vi "Write Core UI References.vi"(8 "error in (no error)":errorcluster, 10 "UI References":T1, 11 "CIF_UI in":refnum<class "CIF_UI.lvclass">) -> (0 "error out":errorcluster, 3 "CIF_UI out":refnum<class "CIF_UI.lvclass">)   [LabVIEW 2021, in "CIF_UI.lvclass"]
uses:
  CIF_UI.lvclass
  Typedef/Core UI References.ctl
  Typedef/Channel Connection.ctl
  Typedef/New Plugin.ctl
  Typedef/Run Listen Button.ctl
  Typedef/CIF_Manager_UI_Tab.ctl
  CIF_UI.lvclass/CIF_UI.ctl
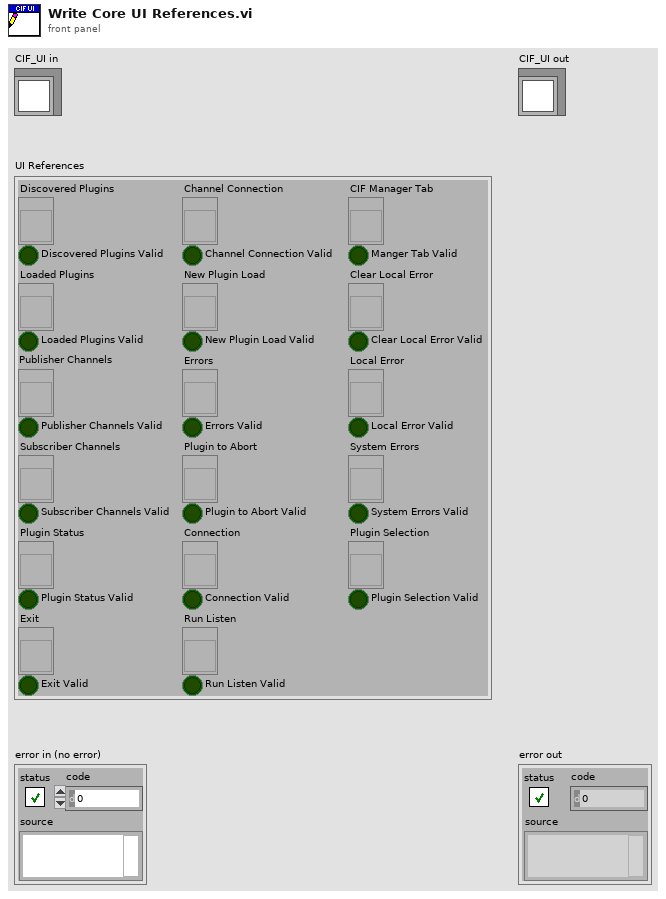
[diagram p1: front panel]
types:
  T1 = typedef "CIF_UI.lvclass/Core UI References.ctl" = cluster{"Discovered Plugins":refnum<vi>, "Discovered Plugins Valid":bool, "Loaded Plugins":refnum<vi>, "Loaded Plugins Valid":bool, "Publisher Channels":refnum<vi>, "Publisher Channels Valid":bool, "Subscriber Channels":refnum<vi>, "Subscriber Channels Valid":bool, "Plugin Status":refnum<vi>, "Plugin Status Valid":bool, "Channel Connection":refnum<vi>, "Channel Connection Valid":bool, "New Plugin Load":refnum<vi>, "New Plugin Load Valid":bool, "Errors":refnum<vi>, "Errors Valid":bool, "Plugin to Abort":refnum<vi>, "Plugin to Abort Valid":bool, "Connection":refnum<vi>, "Connection Valid":bool, "Exit":refnum<vi>, "Exit Valid":bool, "Run Listen":refnum<vi>, "Run Listen Valid":bool, "CIF Manager Tab":refnum<vi>, "Manger Tab Valid":bool, "Clear Local Error":refnum<vi>, "Clear Local Error Valid":bool, "Local Error":refnum<vi>, "Local Error Valid":bool, "System Errors":refnum<vi>, "System Errors Valid":bool, "Plugin Selection":refnum<vi>, "Plugin Selection Valid":bool}
  T2 = typedef "CIF_UI.lvclass/Channel Connection.ctl" = cluster{"Subscriber Name":string, "Publisher Name":string, "Custom Data":string, "FIFO Overrides":cluster{"Backpressure":bool, "Bytes/Message":u32, "Messages/FIFO":u32}}
  T3 = typedef "CIF_UI.lvclass/New Plugin.ctl" = cluster{"Unique Name":string, "Type":string, "Version (Optional)":string}
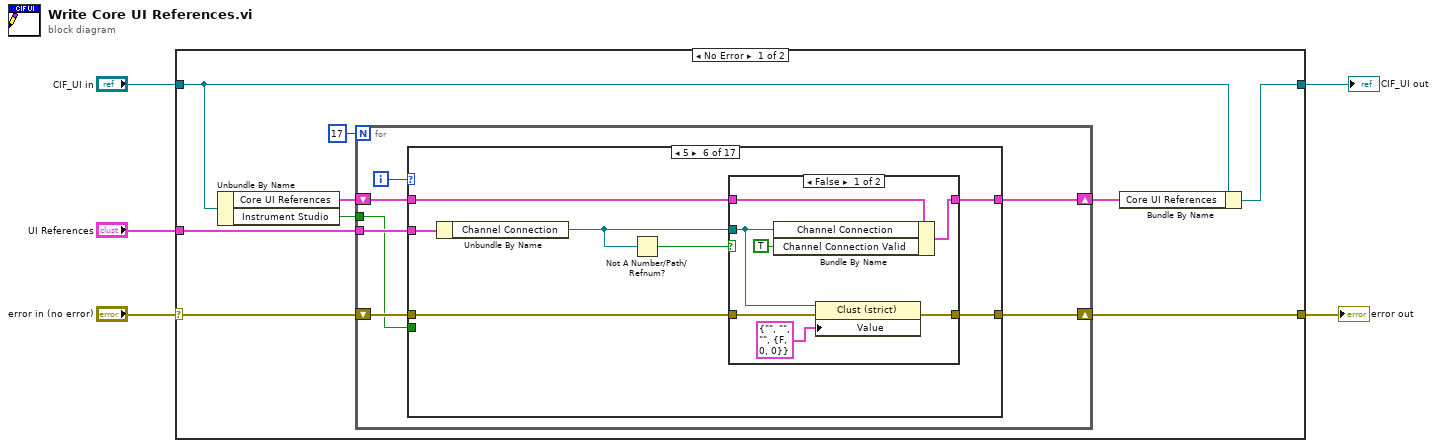
[diagram p0: block diagram]
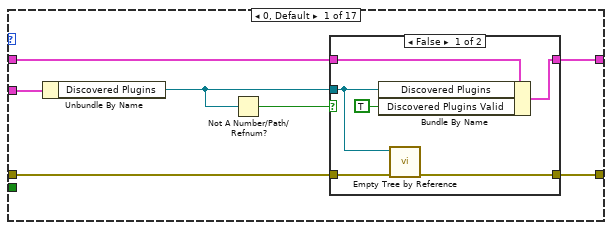
[diagram p2: hidden frame]
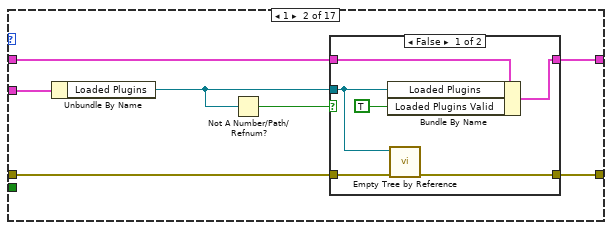
[diagram p4: hidden frame]
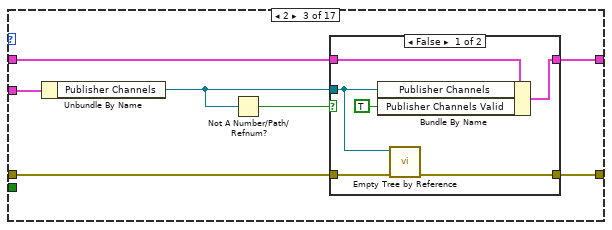
[diagram p6: hidden frame]
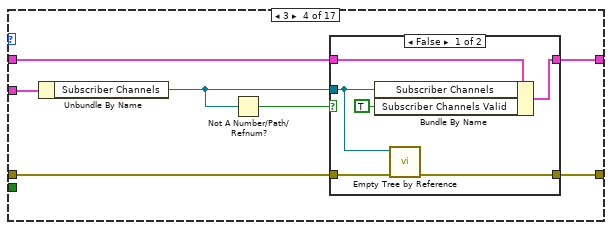
[diagram p8: hidden frame]
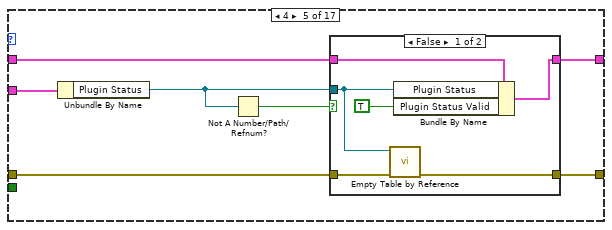
[diagram p10: hidden frame]
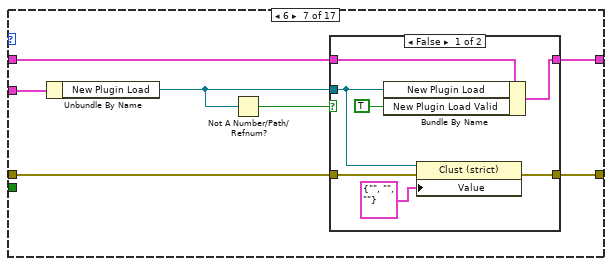
[diagram p13: hidden frame]
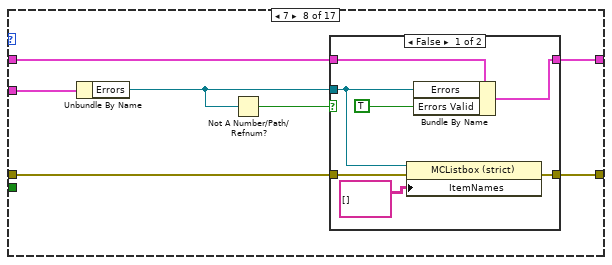
[diagram p15: hidden frame]
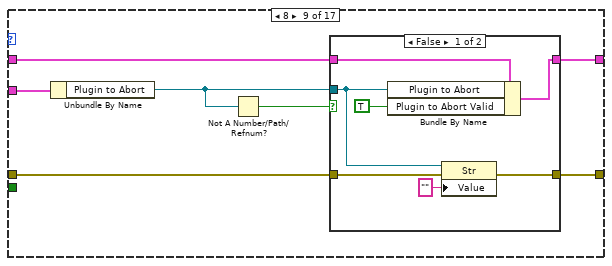
[diagram p17: hidden frame]
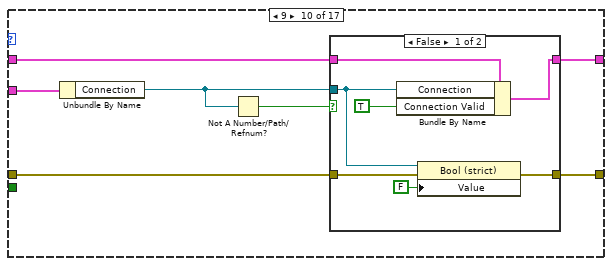
[diagram p19: hidden frame]
diagram:
  n1 = case shown="No Error" "error in (no error)" {
    selector: "error in (no error)" -> [w8 w284]
    tunnel: [w7 w284] -> w4
    tunnel: [w14 w285] -> w2
    tunnel: "CIF_UI in" -> [w12 w285]
    tunnel: "UI References" -> [w13 _]
    frame No Error {
      n2 = Unbundle By Name(w12) -> ("Core UI References"=w11:T1, "Instrument Studio"=w6:bool)
      n3 = for {
        N: 17 -> [_]
        shift-right: [w18] -> w10
        shift-left: w11 -> [w19]
        tunnel: w13 -> [w20]
        shift-right: [w16] -> w7
        shift-left: w8 -> [w17]
        tunnel: w6 -> [w15]
        i -> [w21]
        n4 = case shown="5" w21 {
          tunnel: w20 -> [w28 w43 w58 w73 w88 w103 w119 w135 w151 w167 w184 w201 w217 w232 w246 w262 w276]
          tunnel: w19 -> [w27 w42 w57 w72 w87 w102 w118 w134 w150 w166 w183 w200 w216 w231 w245 w261 w275]
          tunnel: [w26 w41 w56 w71 w86 w101 w117 w133 w149 w165 w182 w199 w215 w230 w244 w260 w274] -> w18
          tunnel: w17 -> [w23 w38 w53 w68 w83 w97 w113 w129 w145 w161 w178 w195 w211 w226 w240 w256 w270]
          tunnel: [w22 w37 w52 w67 w82 w98 w114 w130 w146 w162 w179 w196 w212 w227 w241 w257 w271] -> w16
          tunnel: w15 -> [_ _ _ _ _ _ _ _ _ _ w177 _ _ _ _ _ _]
          frame 0, Default {
            n5 = Unbundle By Name(w28) -> ("Discovered Plugins"=w25:refnum<vi>)
            n6 = Not A Number/Path/Refnum?(number/path/refnum=w25) -> (NaN/Path/Refnum?=w24:bool)
            n7 = case shown="False" w24 {
              tunnel: w25 -> [w31 _]
              tunnel: w27 -> [w34 w36]
              tunnel: [w33 w36] -> w26
              tunnel: w23 -> [w30 w35]
              tunnel: [w29 w35] -> w22
              frame False {
                n8 = Bundle By Name(cluster=w34, "Discovered Plugins"=w31, "Discovered Plugins Valid"=TRUE) -> (w33:T1)
                n9 = call "Empty Tree by Reference.vi"("error in (no error)"=w30, "Tree ref in"=w31) -> ("error out"=w29:errorcluster)  [unwired: 9 in]
              }
              frame True {
              }
            }
          }
          frame 1 {
            n10 = Unbundle By Name(w43) -> ("Loaded Plugins"=w40:refnum<vi>)
            n11 = Not A Number/Path/Refnum?(number/path/refnum=w40) -> (NaN/Path/Refnum?=w39:bool)
            n12 = case shown="False" w39 {
              tunnel: w40 -> [w46 _]
              tunnel: w42 -> [w49 w51]
              tunnel: [w48 w51] -> w41
              tunnel: w38 -> [w45 w50]
              tunnel: [w44 w50] -> w37
              frame False {
                n13 = Bundle By Name(cluster=w49, "Loaded Plugins"=w46, "Loaded Plugins Valid"=TRUE ("Discovered Plugins Valid")) -> (w48:T1)
                n14 = call "Empty Tree by Reference.vi"("error in (no error)"=w45, "Tree ref in"=w46) -> ("error out"=w44:errorcluster)  [unwired: 9 in]
              }
              frame True {
              }
            }
          }
          frame 2 {
            n15 = Unbundle By Name(w58) -> ("Publisher Channels"=w55:refnum<vi>)
            n16 = Not A Number/Path/Refnum?(number/path/refnum=w55) -> (NaN/Path/Refnum?=w54:bool)
            n17 = case shown="False" w54 {
              tunnel: w55 -> [w61 _]
              tunnel: w57 -> [w64 w66]
              tunnel: [w63 w66] -> w56
              tunnel: w53 -> [w60 w65]
              tunnel: [w59 w65] -> w52
              frame False {
                n18 = Bundle By Name(cluster=w64, "Publisher Channels"=w61, "Publisher Channels Valid"=TRUE ("Discovered Plugins Valid")) -> (w63:T1)
                n19 = call "Empty Tree by Reference.vi"("error in (no error)"=w60, "Tree ref in"=w61) -> ("error out"=w59:errorcluster)  [unwired: 9 in]
              }
              frame True {
              }
            }
          }
          frame 3 {
            n20 = Unbundle By Name(w73) -> ("Subscriber Channels"=w70:refnum<vi>)
            n21 = Not A Number/Path/Refnum?(number/path/refnum=w70) -> (NaN/Path/Refnum?=w69:bool)
            n22 = case shown="False" w69 {
              tunnel: w70 -> [w76 _]
              tunnel: w72 -> [w79 w81]
              tunnel: [w78 w81] -> w71
              tunnel: w68 -> [w75 w80]
              tunnel: [w74 w80] -> w67
              frame False {
                n23 = Bundle By Name(cluster=w79, "Subscriber Channels"=w76, "Subscriber Channels Valid"=TRUE ("Discovered Plugins Valid")) -> (w78:T1)
                n24 = call "Empty Tree by Reference.vi"("error in (no error)"=w75, "Tree ref in"=w76) -> ("error out"=w74:errorcluster)  [unwired: 9 in]
              }
              frame True {
              }
            }
          }
          frame 4 {
            n25 = Unbundle By Name(w88) -> ("Plugin Status"=w85:refnum<vi>)
            n26 = Not A Number/Path/Refnum?(number/path/refnum=w85) -> (NaN/Path/Refnum?=w84:bool)
            n27 = case shown="False" w84 {
              tunnel: w85 -> [w90 _]
              tunnel: w87 -> [w94 w96]
              tunnel: [w93 w96] -> w86
              tunnel: w83 -> [w91 w95]
              tunnel: [w89 w95] -> w82
              frame False {
                n28 = call "Empty Table by Reference.vi"("error in (no error)"=w91, "Table Control in"=w90) -> ("error out"=w89:errorcluster)  [unwired: 9 in]
                n29 = Bundle By Name(cluster=w94, "Plugin Status"=w90, "Plugin Status Valid"=TRUE ("Discovered Plugins Valid")) -> (w93:T1)
              }
              frame True {
              }
            }
          }
          frame 5 {
            n30 = Unbundle By Name(w103) -> ("Channel Connection"=w100:refnum<vi>)
            n31 = Not A Number/Path/Refnum?(number/path/refnum=w100) -> (NaN/Path/Refnum?=w99:bool)
            n32 = case shown="False" w99 {
              tunnel: w100 -> [w107 _]
              tunnel: w102 -> [w110 w112]
              tunnel: [w109 w112] -> w101
              tunnel: [w106 w111] -> w98
              tunnel: w97 -> [w105 w111]
              frame False {
                n33 = Bundle By Name(cluster=w110, "Channel Connection"=w107, "Channel Connection Valid"=TRUE ("Discovered Plugins Valid")) -> (w109:T1)
                n34 = property on="Property Node" class="Clust (strict)"(reference=w107, error in=w105, "Value"=T2 {"Subscriber Name"="", "Publisher Name"="", "Custom Data"="", "FIFO Overrides"={"Backpressure"=FALSE, "Bytes/Message"=0, "Messages/FIFO"=0}}) -> (error out=w106:errorcluster)  [unwired: 1 out]
              }
              frame True {
              }
            }
          }
          frame 6 {
            n35 = Unbundle By Name(w119) -> ("New Plugin Load"=w116:refnum<vi>)
            n36 = Not A Number/Path/Refnum?(number/path/refnum=w116) -> (NaN/Path/Refnum?=w115:bool)
            n37 = case shown="False" w115 {
              tunnel: w116 -> [w123 _]
              tunnel: w118 -> [w126 w128]
              tunnel: [w125 w128] -> w117
              tunnel: [w122 w127] -> w114
              tunnel: w113 -> [w121 w127]
              frame False {
                n38 = Bundle By Name(cluster=w126, "New Plugin Load"=w123, "New Plugin Load Valid"=TRUE ("Discovered Plugins Valid")) -> (w125:T1)
                n39 = property on="Property Node" class="Clust (strict)"(reference=w123, error in=w121, "Value"=T3 {"Unique Name"="", "Type"="", "Version (Optional)"=""}) -> (error out=w122:errorcluster)  [unwired: 1 out]
              }
              frame True {
              }
            }
          }
          frame 7 {
            n40 = Unbundle By Name(w135) -> ("Errors"=w132:refnum<vi>)
            n41 = Not A Number/Path/Refnum?(number/path/refnum=w132) -> (NaN/Path/Refnum?=w131:bool)
            n42 = case shown="False" w131 {
              tunnel: w132 -> [w139 _]
              tunnel: w134 -> [w142 w144]
              tunnel: [w141 w144] -> w133
              tunnel: [w138 w143] -> w130
              tunnel: w129 -> [w137 w143]
              frame False {
                n43 = property on="Property Node" class="MCListbox (strict)"(reference=w139, error in=w137, "ItemNames"=string[][] [] ("Item Names")) -> (error out=w138:errorcluster)  [unwired: 1 out]
                n44 = Bundle By Name(cluster=w142, "Errors"=w139, "Errors Valid"=TRUE ("Discovered Plugins Valid")) -> (w141:T1)
              }
              frame True {
              }
            }
          }
          frame 8 {
            n45 = Unbundle By Name(w151) -> ("Plugin to Abort"=w148:refnum<vi>)
            n46 = Not A Number/Path/Refnum?(number/path/refnum=w148) -> (NaN/Path/Refnum?=w147:bool)
            n47 = case shown="False" w147 {
              tunnel: w148 -> [w155 _]
              tunnel: w150 -> [w158 w160]
              tunnel: [w157 w160] -> w149
              tunnel: [w154 w159] -> w146
              tunnel: w145 -> [w153 w159]
              frame False {
                n48 = Bundle By Name(cluster=w158, "Plugin to Abort"=w155, "Plugin to Abort Valid"=TRUE ("Discovered Plugins Valid")) -> (w157:T1)
                n49 = property on="Property Node" class="Str"(reference=w155, error in=w153, "Value"="") -> (error out=w154:errorcluster)  [unwired: 1 out]
              }
              frame True {
              }
            }
          }
          frame 9 {
            n50 = Unbundle By Name(w167) -> ("Connection"=w164:refnum<vi>)
            n51 = Not A Number/Path/Refnum?(number/path/refnum=w164) -> (NaN/Path/Refnum?=w163:bool)
            n52 = case shown="False" w163 {
              tunnel: w164 -> [w171 _]
              tunnel: w166 -> [w174 w176]
              tunnel: [w173 w176] -> w165
              tunnel: [w170 w175] -> w162
              tunnel: w161 -> [w169 w175]
              frame False {
                n53 = Bundle By Name(cluster=w174, "Connection"=w171, "Connection Valid"=TRUE ("Discovered Plugins Valid")) -> (w173:T1)
                n54 = property on="Property Node" class="Bool (strict)"(reference=w171, error in=w169, "Value"=FALSE) -> (error out=w170:errorcluster)  [unwired: 1 out]
              }
              frame True {
              }
            }
          }
          frame 10 {
            n55 = Unbundle By Name(w184) -> ("Exit"=w181:refnum<vi>)
            n56 = Not A Number/Path/Refnum?(number/path/refnum=w181) -> (NaN/Path/Refnum?=w180:bool)
            n57 = case shown="False" w180 {
              tunnel: w181 -> [w189 _]
              tunnel: w183 -> [w192 w194]
              tunnel: [w191 w194] -> w182
              tunnel: [w188 w193] -> w179
              tunnel: w178 -> [w187 w193]
              tunnel: w177 -> [w186 _]
              frame False {
                n58 = Not(x=w186) -> (.not. x?=w185:bool)
                n59 = Bundle By Name(cluster=w192, "Exit"=w189, "Exit Valid"=TRUE ("Discovered Plugins Valid")) -> (w191:T1)
                n60 = property on="Property Node" class="Bool"(reference=w189, error in=w187, "Visible"=w185) -> (error out=w188:errorcluster)  [unwired: 1 out]
              }
              frame True {
              }
            }
          }
          frame 11 {
            n61 = Unbundle By Name(w201) -> ("Run Listen"=w198:refnum<vi>)
            n62 = Not A Number/Path/Refnum?(number/path/refnum=w198) -> (NaN/Path/Refnum?=w197:bool)
            n63 = case shown="False" w197 {
              tunnel: w198 -> [w205 _]
              tunnel: w200 -> [w208 w210]
              tunnel: [w207 w210] -> w199
              tunnel: [w204 w209] -> w196
              tunnel: w195 -> [w203 w209]
              frame False {
                n64 = Bundle By Name(cluster=w208, "Run Listen"=w205, "Run Listen Valid"=TRUE ("Discovered Plugins Valid")) -> (w207:T1)
                n65 = property on="Property Node" class="Bool"(reference=w205, error in=w203, "Value"=FALSE) -> (error out=w204:errorcluster)  [unwired: 1 out]
              }
              frame True {
              }
            }
          }
          frame 12 {
            n66 = Unbundle By Name(w217) -> ("CIF Manager Tab"=w214:refnum<vi>)
            n67 = Not A Number/Path/Refnum?(number/path/refnum=w214) -> (NaN/Path/Refnum?=w213:bool)
            n68 = case shown="False" w213 {
              tunnel: w214 -> [w218 _]
              tunnel: w216 -> [w223 w225]
              tunnel: [w222 w225] -> w215
              tunnel: [w219 w224] -> w212
              tunnel: w211 -> [w220 w224]
              frame False {
                n69 = Bundle By Name(cluster=w223, "CIF Manager Tab"=w218, "Manger Tab Valid"=TRUE ("Discovered Plugins Valid")) -> (w222:T1)
                n70 = call "Initialize Manager Tab by Reference.vi"("error in (no error)"=w220, "CIF Manager UI Tab"=w218) -> ("error out"=w219:errorcluster)  [unwired: 9 in]
              }
              frame True {
              }
            }
          }
          frame 13 {
            n71 = Unbundle By Name(w232) -> ("Clear Local Error"=w229:refnum<vi>)
            n72 = Not A Number/Path/Refnum?(number/path/refnum=w229) -> (NaN/Path/Refnum?=w228:bool)
            n73 = case shown="False" w228 {
              tunnel: w229 -> [w234 _]
              tunnel: w231 -> [w237 w239]
              tunnel: [w236 w239] -> w230
              tunnel: [w233 w238] -> w227
              tunnel: w226 -> [w233 w238]
              frame False {
                n74 = Bundle By Name(cluster=w237, "Clear Local Error"=w234, "Clear Local Error Valid"=TRUE ("Discovered Plugins Valid")) -> (w236:T1)
              }
              frame True {
              }
            }
          }
          frame 14 {
            n75 = Unbundle By Name(w246) -> ("Local Error"=w243:refnum<vi>)
            n76 = Not A Number/Path/Refnum?(number/path/refnum=w243) -> (NaN/Path/Refnum?=w242:bool)
            n77 = case shown="False" w242 {
              tunnel: w243 -> [w249 _]
              tunnel: w245 -> [w253 w255]
              tunnel: [w252 w255] -> w244
              tunnel: [w247 w254] -> w241
              tunnel: w240 -> [w248 w254]
              frame False {
                n78 = Bundle By Name(cluster=w253, "Local Error"=w249, "Local Error Valid"=TRUE ("Discovered Plugins Valid")) -> (w252:T1)
                n79 = property on="Property Node" class="Str"(reference=w249, error in=w248, "Value"="") -> (error out=w247:errorcluster)  [unwired: 1 out]
              }
              frame True {
              }
            }
          }
          frame 15 {
            n80 = Unbundle By Name(w262) -> ("System Errors"=w259:refnum<vi>)
            n81 = Not A Number/Path/Refnum?(number/path/refnum=w259) -> (NaN/Path/Refnum?=w258:bool)
            n82 = case shown="False" w258 {
              tunnel: w259 -> [w264 _]
              tunnel: w261 -> [w267 w269]
              tunnel: [w266 w269] -> w260
              tunnel: [w263 w268] -> w257
              tunnel: w256 -> [w263 w268]
              frame False {
                n83 = Bundle By Name(cluster=w267, "System Errors"=w264, "System Errors Valid"=TRUE ("Discovered Plugins Valid")) -> (w266:T1)
              }
              frame True {
              }
            }
          }
          frame 16 {
            n84 = Unbundle By Name(w276) -> ("Plugin Selection"=w273:refnum<vi>)
            n85 = Not A Number/Path/Refnum?(number/path/refnum=w273) -> (NaN/Path/Refnum?=w272:bool)
            n86 = case shown="False" w272 {
              tunnel: w273 -> [w278 _]
              tunnel: w275 -> [w281 w283]
              tunnel: [w280 w283] -> w274
              tunnel: [w277 w282] -> w271
              tunnel: w270 -> [w277 w282]
              frame False {
                n87 = Bundle By Name(cluster=w281, "Plugin Selection"=w278, "Plugin Selection Valid"=TRUE ("Discovered Plugins Valid")) -> (w280:T1)
              }
              frame True {
              }
            }
          }
        }
      }
      n88 = Bundle By Name(cluster=w12, "Core UI References"=w10) -> (w14:refnum<class "CIF_UI.lvclass">)
    }
    frame Error {
    }
  }
  "error out" <- w4
  "CIF_UI out" <- w2
